vi "Read All Control Values.vi"(8 "error in (no error)":errorcluster, 11 "CD Parameter Manager in":refnum<class "CD Parameter Manager.lvclass">) -> (0 "error out":errorcluster, 3 "CD Parameter Manager out":refnum<class "CD Parameter Manager.lvclass">)   [LabVIEW 2016, in "CD Parameter Manager API.lvlib" / "CD Parameter Manager.lvclass"]
uses:
  CD Parameter Manager.lvclass
  Parameter Class/Parameter.lvclass
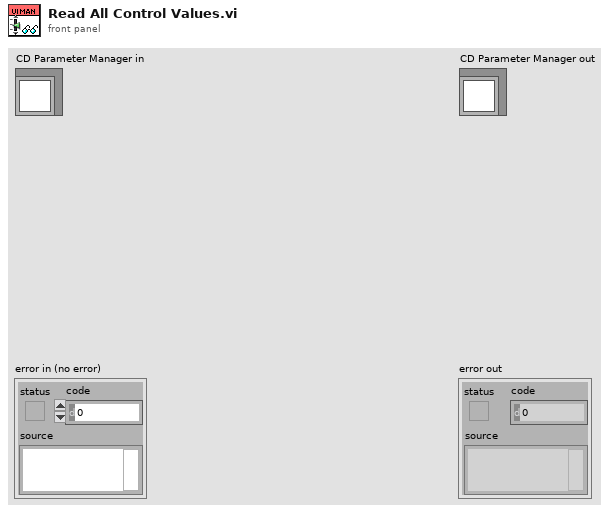
[diagram p1: front panel]
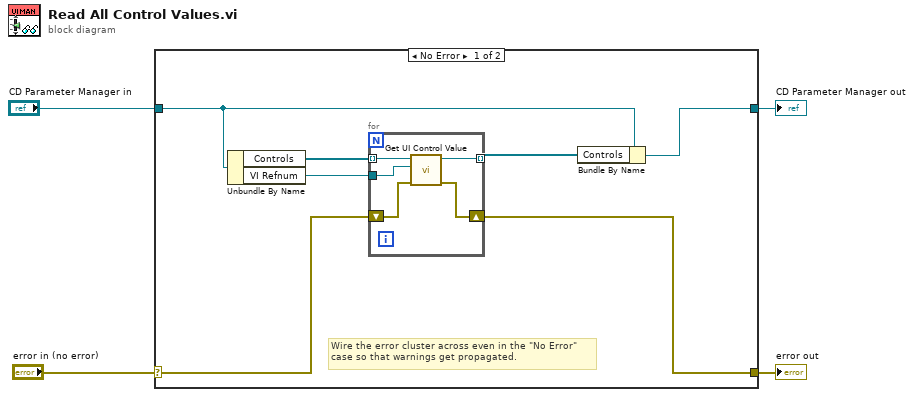
[diagram p0: block diagram]
diagram:
  n1 = case shown="No Error" "error in (no error)" {
    selector: "error in (no error)" -> [w9 w18]
    tunnel: [w8 w18] -> w3
    tunnel: [w5 w17] -> w1
    tunnel: "CD Parameter Manager in" -> [w6 w17]
    frame No Error {
      # "Wire the error cluster across even in the \"No Error\"\ncase so that warnings get propagated."
      n2 = Unbundle By Name(w6) -> ("Controls"=w10:refnum<class "Parameter.lvclass">[], "VI Refnum"=w11:refnum<vi>)
      n3 = for {
        tunnel: w11 -> [w16]
        tunnel: w10 -> [w15] mode=indexing
        shift-right: [w13] -> w8
        shift-left: w9 -> [w14]
        tunnel: [w12] -> w7 mode=indexing
        n4 = call-dynamic "Get UI Control Value.vi"("error in (no error)"=w14, "VI Ref"=w16, "Parameter in"=w15) -> ("error out"=w13:errorcluster, "Parameter out"=w12:refnum<class "Parameter.lvclass">)  [unwired: 7 in]
      }
      n5 = Bundle By Name(cluster=w6, "Controls"=w7) -> (w5:refnum<class "CD Parameter Manager.lvclass">)
    }
    frame Error {
    }
  }
  "error out" <- w3
  "CD Parameter Manager out" <- w1
